vi "Test Find Value.vi"() -> ()   [LabVIEW 2020]
uses:
  Test Type A/Test Type A.lvclass
  Test Type B.lvclass
  PathTree/PathTree/PathTree.lvclass
panel:
  out "Data":variant
  out "class name":string
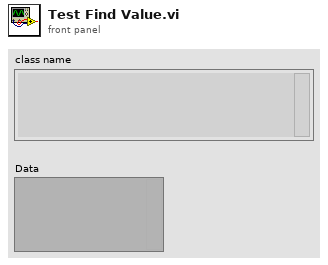
[diagram p1: front panel]
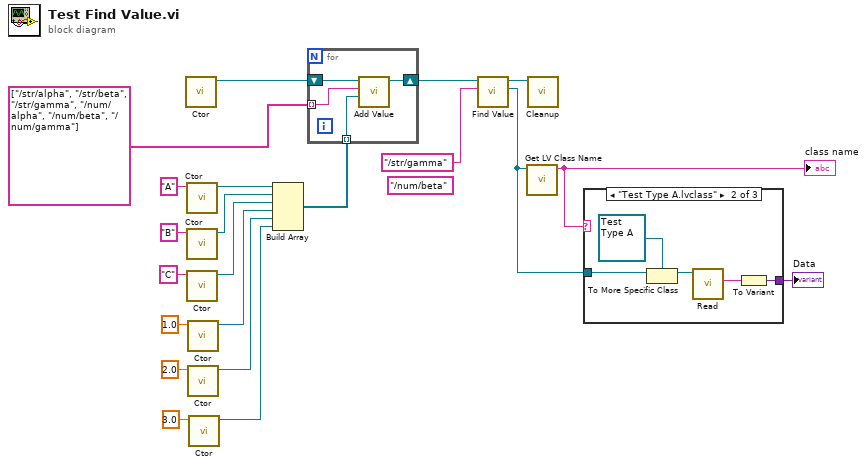
[diagram p0: block diagram]
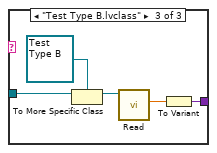
[diagram p3: hidden frame]
diagram:
  (unwired) "/num/beta"
  n1 = call "Ctor.vi"() -> ("PathTree out"=w15:refnum<class "PathTree.lvclass">)  [unwired: 10 in, 1 out]
  n2 = call "Ctor.vi"("Value"="A") -> ("Test Type A out"=w14:refnum<class "Test Type A.lvclass">)  [unwired: 9 in, 1 out]
  n3 = call "Ctor.vi"("Value"="B") -> ("Test Type A out"=w13:refnum<class "Test Type A.lvclass">)  [unwired: 9 in, 1 out]
  n4 = call "Ctor.vi"("Value"="C") -> ("Test Type A out"=w12:refnum<class "Test Type A.lvclass">)  [unwired: 9 in, 1 out]
  n5 = call "Ctor.vi"("Value"=1.0) -> ("Test Type B out"=w11:refnum<class "Test Type B.lvclass">)  [unwired: 9 in, 1 out]
  n6 = call "Ctor.vi"("Value"=2.0) -> ("Test Type B out"=w10:refnum<class "Test Type B.lvclass">)  [unwired: 9 in, 1 out]
  n7 = call "Ctor.vi"("Value"=3.0) -> ("Test Type B out"=w9:refnum<class "Test Type B.lvclass">)  [unwired: 9 in, 1 out]
  n8 = Build Array(w14, w13, w12, w11, w10, w9) -> (w8:refnum<class>[])
  n9 = for {
    tunnel: w8 -> [w24] mode=indexing
    tunnel: string[] ["/str/alpha", "/str/beta", "/str/gamma", "/num/alpha", "/num/beta", "/num/gamma"] -> [w23] mode=indexing
    shift-right: [w22] -> w6
    shift-left: w15 -> [w25]
    n10 = call "Add Value.vi"("Value"=w24, "Path"=w23, "PathTree in"=w25) -> ("PathTree out"=w22:refnum<class "PathTree.lvclass">)  [unwired: 7 in, 1 out]
  }
  n11 = call "Find Value.vi"("Path"="/str/gamma", "PathTree in"=w6) -> ("Value"=w3:refnum<class>, "PathTree out"=w5:refnum<class "PathTree.lvclass">)  [unwired: 7 in, 1 out]
  n12 = call <vilib>:"Get LV Class Name.vi"("object"=w3) -> ("class name"=w4:string)  [unwired: 9 in, 1 out]
  "class name" <- w4
  n13 = call "Cleanup.vi"("PathTree in"=w5) -> ()  [unwired: 10 in, 1 out]
  n14 = case shown="\"Test Type A.lvclass\"" w4 {
    tunnel: w3 -> [_ w30 w35]
    tunnel: [_ w26 w34] -> w2
    frame Default {
    }
    frame "Test Type A.lvclass" {
      n15 = To More Specific Class(target class=refnum<class "Test Type A.lvclass"> refnum ("Test Type A.lvclass"), reference=w30) -> (specific class reference=w28:refnum<class "Test Type A.lvclass">)  [unwired: 1 in, 1 out]
      n16 = call "Read.vi"("Test Type A in"=w28) -> ("Value"=w27:string)  [unwired: 8 in, 2 out]
      n17 = To Variant(anything=w27) -> (Variant=w26:variant)
    }
    frame "Test Type B.lvclass" {
      n18 = To More Specific Class(target class=refnum<class "Test Type B.lvclass"> refnum ("Test Type B.lvclass"), reference=w35) -> (specific class reference=w32:refnum<class "Test Type B.lvclass">)  [unwired: 1 in, 1 out]
      n19 = call "Read.vi"("Test Type B in"=w32) -> ("Value"=w31:dbl)  [unwired: 8 in, 2 out]
      n20 = To Variant(anything=w31) -> (Variant=w34:variant)
    }
  }
  "Data" <- w2
